vi "tearDown.vi"(8 "error in (no error)":errorcluster, 11 "reference in":refnum<class "Routing and Faulting Import Unit Tests.lvclass">) -> (0 "error out":errorcluster, 3 "reference out":refnum<class "Routing and Faulting Import Unit Tests.lvclass">)   [LabVIEW 2019, in "Routing and Faulting Import Unit Tests.lvclass"]
doc: "tearDown runs after the test method has completed. Use this method to clean up any operations or references that were opened by setUp or the test method. Unit tests should be independent of other unit tests so this VI should ensure that the next test can run in a 'clean' test environment."
uses:
  Routing and Faulting Import Unit Tests.lvclass
  Routing and Faulting Import Unit Tests.lvclass/Routing and Faulting Import Unit Tests.ctl
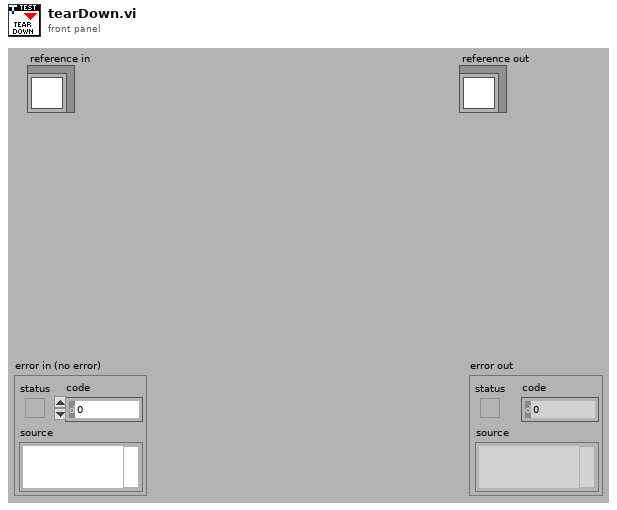
[diagram p1: front panel]
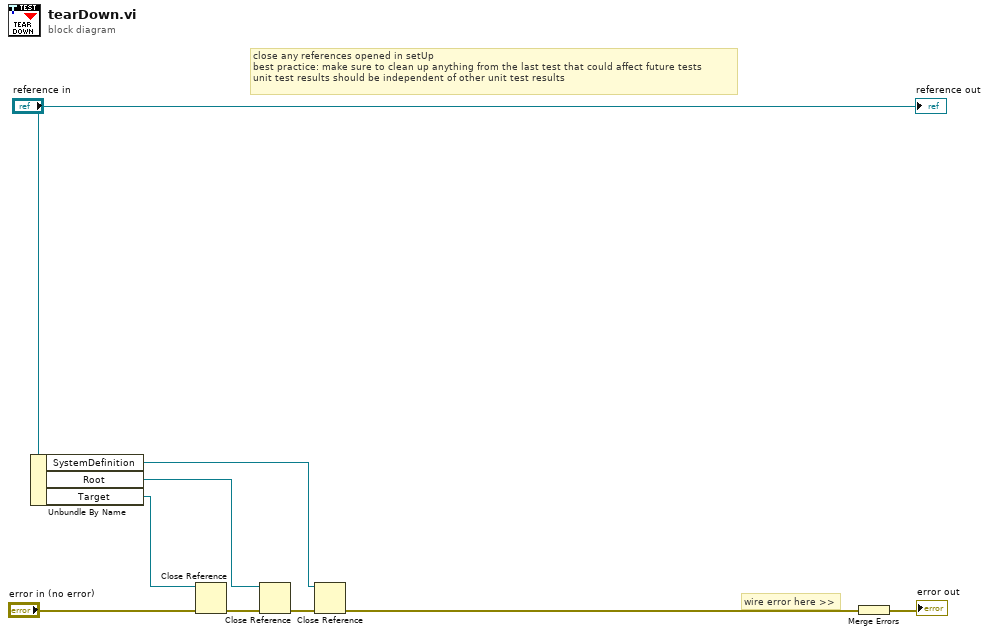
[diagram p0: block diagram]
diagram:
  # "wire error here >>"
  # "close any references opened in setUp\nbest practice: make sure to clean up anything from the last test that could affect future tests\nunit test results should be independent of other unit test results"
  n1 = Unbundle By Name("reference in") -> ("SystemDefinition"=w2:refnum<k24>, "Root"=w4:refnum<k24>, "Target"=w6:refnum<k24>)
  n2 = Close Reference(reference=w6, error in (no error)="error in (no error)") -> (error out=w5:errorcluster)
  n3 = Close Reference(reference=w4, error in (no error)=w5) -> (error out=w3:errorcluster)
  n4 = Close Reference(reference=w2, error in (no error)=w3) -> (error out=w1:errorcluster)
  n5 = Merge Errors(w1) -> (→"error out":errorcluster)
  "reference out" <- "reference in"
